vi "Global_SEN_Data Out.vi"() -> ()   [LabVIEW 2020, in "Swerve_Odometry_SEN.lvlib"]
uses:
  Swerve_Odometry_SEN.lvlib
  Cluster_SWERVE_DRIVE_ODOMETRY.ctl
  Cluster_POSE2D.ctl
  Cluster_TRANSLATION2D.ctl
  Cluster_ROTATION2D.ctl
  Cluster_SWERVE_DRIVE_MODULE_POSITION.ctl
panel:
  out "SEN_SWERVE_DRIVE_ODOMETRY_Values":T1={"POSE"={"TRANSLATION"={"X"=0.0, "Y"=0.0}, "ROTATION"={"VALUE"=0.0, "COS"=1.0, "SIN"=0.0}}, "GyroOffset"={"VALUE"=0.0, "COS"=1.0, "SIN"=0.0}, "PreviousAngle"={"VALUE"=0.0, "COS"=1.0, "SIN"=0.0}, "PrevTime"=0.0, "PrevModulePosition"=[], "NumModules"=0} {"PrevModulePosition"."Angle"."SIN" format="%13.4f"; "PrevModulePosition"."Angle"."COS" format="%13.4f"; "PrevModulePosition"."Angle"."VALUE" format="%13.4f"; "PreviousAngle"."SIN" format="%13.4f"; "PreviousAngle"."COS" format="%13.4f"; "PreviousAngle"."VALUE" format="%13.4f"; "GyroOffset"."SIN" format="%13.4f"; "GyroOffset"."COS" format="%13.4f"; "GyroOffset"."VALUE" format="%13.4f"; "POSE"."ROTATION"."SIN" format="%13.4f"; "POSE"."ROTATION"."COS" format="%13.4f"; "POSE"."ROTATION"."VALUE" format="%13.4f"; "POSE"."TRANSLATION"."Y" format="%14.3f"; "POSE"."TRANSLATION"."X" format="%14.3f"}
  in  "SEN_Is_Tracking":bool
  in  "SEN_Template_CycleTime(S)":dbl
  # "The Names of the Data items in the Global Variable MUST describe who the Single Writer is\nFor Sensor Globals the the naming convention is\n   \nSEN_Lib Name_Data Name\n\nExamples:\nSEN_Gyro_Angle\nSEN_Sonar_Distance"
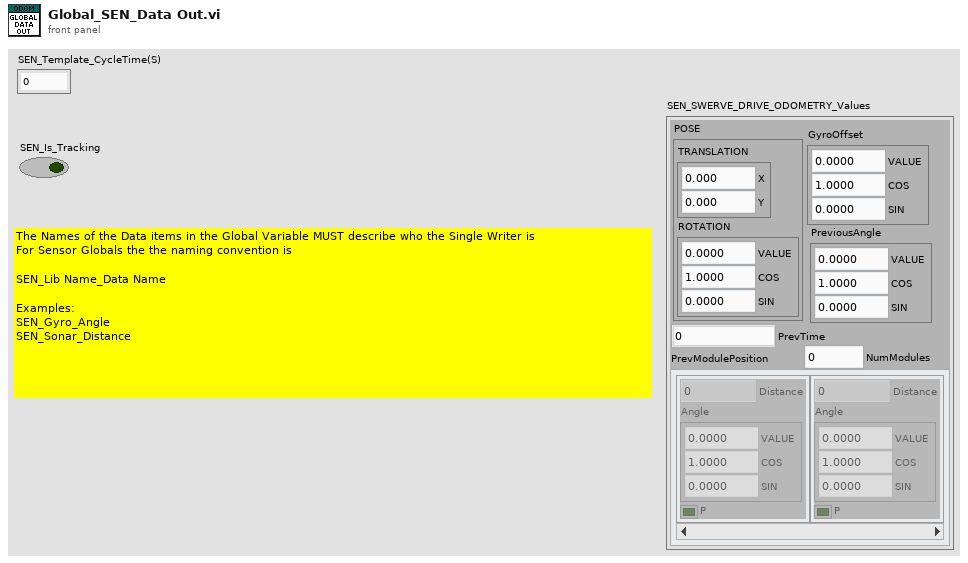
[diagram p1: front panel]
types:
  T1 = typedef "Swerve_Odometry_SEN.lvlib/Cluster_SWERVE_DRIVE_ODOMETRY.ctl" = cluster{"POSE":T2, "GyroOffset":T4, "PreviousAngle":T4, "PrevTime":dbl, "PrevModulePosition":T5[], "NumModules":i32}
  T2 = typedef "Swerve_Odometry_SEN.lvlib/Cluster_POSE2D.ctl" = cluster{"TRANSLATION":T3, "ROTATION":T4}
  T3 = typedef "Swerve_Odometry_SEN.lvlib/Cluster_TRANSLATION2D.ctl" = cluster{"X":dbl, "Y":dbl}
  T4 = typedef "Swerve_Odometry_SEN.lvlib/Cluster_ROTATION2D.ctl" = cluster{"VALUE":dbl, "COS":dbl, "SIN":dbl}
  T5 = typedef "Swerve_Odometry_SEN.lvlib/Cluster_SWERVE_DRIVE_MODULE_POSITION.ctl" = cluster{"Distance":dbl, "Angle":T4, "P":bool}
diagram:
